vi "SingleGUI-Intravital.vi"() -> ()   [LabVIEW 2011]
uses:
  <vilib>/event_ctls.llb/lveventtype.ctl
  <vilib>/Utility/inputDevices.llb/mouseAcquire.vi
  <vilib>/Utility/inputDevices.llb/closeMouse.vi
panel:
  in  "Shutter":bool
  in  "LaserPower mW":dbl(slide) scale=1.0..500.0
  in  "Menu":string
  in  "Intensity":dbl(slide) scale=0.0..5.0
  in  "PMT2 ON":bool=TRUE caption="PMT2"
  in  "High Voltage PMT / V 2":u16(slide) caption="High Voltage PMT2 / V" max=1250 step=1 scale=0.0..1250.0
  in  "Pos [mm]":cluster{"x":dbl, "y":dbl}={"x"=56.550000000000004, "y"=34.7} {"x" min=-200.0 max=200.0 step=0.01 format="%.4f"; "y" min=-100.0 max=100.0 step=0.01 format="%.4f"}
  in  "Stage control":enum32{"xy", "Setup", "Status"}(tab)
  in  "Stepsize [mm]":dbl(slide)=0.4602583962404807 scale=0.01..5.0
  in  "Cluster":T1
  in  "clockwise":bool=TRUE
  in  "xy Angle":dbl
  in  "Objektiv Offsets":cluster{"x":dbl, "y":dbl, "z":dbl}[](array[cluster]) {"z" format="%#.3p"; "y" format="%#.3p"; "x" format="%#.3p"}
  out "scroll units^3":dbl
  out "Mouse inside?":T2
  out "scroll timed out":bool=TRUE
  out "endGUI":bool
  in  "z[mm]":dbl(slide) min=0.0 max=21.5 step=1e-05 scale format="%#.3f"
  in  "PMT Filter":sgl(ring) caption="filter.f1" items=["Split562", "Split495", "empty"]
  in  "Epi Filter":sgl(ring) caption="filter.f2" items=["emty"=0, "empty"=5]
  in  "PMT1 ON":bool=TRUE caption="PMT1"
  in  "High Voltage PMT / V":u16(slide) max=1250 step=1 scale=0.0..1250.0
  in  "stop 2":bool
  in  "continous":bool
  in  "LED":bool
  in  "single":bool
  in  "Camera Exposure (s)":dbl(slide)=0.08565902153685491 min=1e-06 step=0.001 scale=0.001..10.0 scale format="%#.3p"
  in  "Channel1=f":bool
  in  "End Program":bool
  out "Image":T3(plugin-control)
  in  "Detector":u16(ring)
  out "Image Nr":i32
  in  "Conversion Method":u32(ring)=2 items=["Full Dynamic"=0, "Given Range"=2, "90% Dynamic"=3, "Given Percent Range"=4]
  in  "Max. Value":i32=1000 min=1 max=64000 step=50
  in  "Min. Value":i32 min=0 max=32000 step=10
  # "Colibri Laser Scanning                                                                                                                                                 TILL Photonics GmbH"
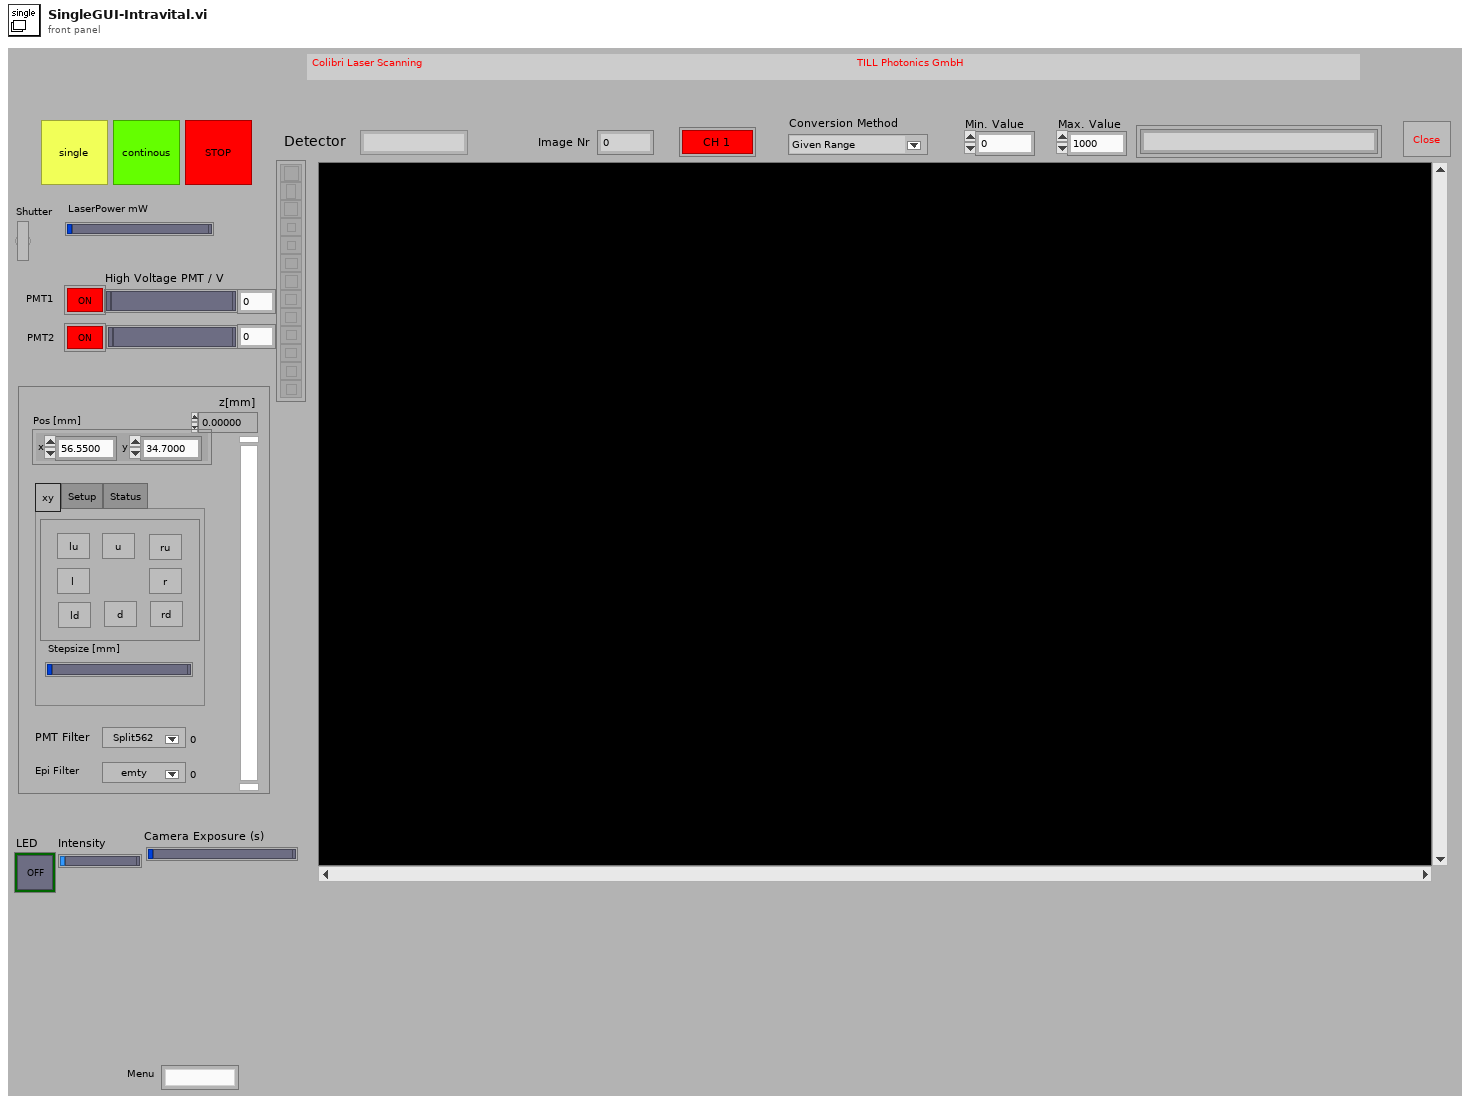
[diagram p1: front panel]
types:
  T1 = cluster{"r":bool, "ru":bool, "u":bool, "lu":bool, "l":bool, "ld":bool, "d":bool, "rd":bool}
  T2 = typedef "lveventtype.ctl" = enum32{"Null", "Timeout", "App Instance Close", "App Instance Close?", "Autoscale Range Change", "Cell Edit", "Cell Edit?", "Cursor Grab", "Cursor Grab?", "Cursor Move", "Cursor Release", "Data Change", "Direction Change", "Display State Change", "Drag Ended", "Drag Enter", "Drag Leave", "Drag Over", "Drag Source Update", "Drag Starting", "Drag Starting?", "Drop", "Exec State Change", "Key Down", "Key Down?", "Key Repeat", "Key Repeat?", "Key Up", "Listbox Double Click", "Menu Activation?", "Menu Selection (App)", "Menu Selection? (App)", "Menu Selection (User)", "Mouse Down", "Mouse Down?", "Mouse Enter", "Mouse Leave", "Mouse Move", "Mouse Up", "NI Security User Change (App)", "Pane Size", "Panel Close", "Panel Close?", "Panel Resize", "Plot Attribute Change", "Scale Range Change", "Shortcut Menu Activation?", "Shortcut Menu Selection (App)", "Shortcut Menu Selection? (App)", "Shortcut Menu Selection (User)", "Tree Double Click", "Tree Drag", "Tree Drag?", "Tree Drop", "Tree Drop?", "Tree Item Close", "Tree Item Close?", "Tree Item Open", "Tree Item Open?", "Value Change"}
  T3 = typedef "IMAQ Image.ctl" = refnum<image>
  T4 = enum16{"None/#Datasets", "Clear", "TagValueOf#", "AddValues", "ReadValue", "ChangeValue", "Get all"}
  T5 = enum16{"status", "createIMAQ", "getIMAQ", "getNumber", "deleteIMAQ", "deleteAll", "MemoryUsage", "GetAccess", "DecreaseAccess", "ActualIndex", "ElementToNumber"}
  T6 = cluster{"default value 1":dbl, "default value 1":dbl, "default value 1":dbl}
  T7 = cluster{"menu tag":string, "menu-vi":refnum<vi>}[]
  T8 = cluster{"Horizontal":i32, "Vertical":i32, "Scrolling":i32}
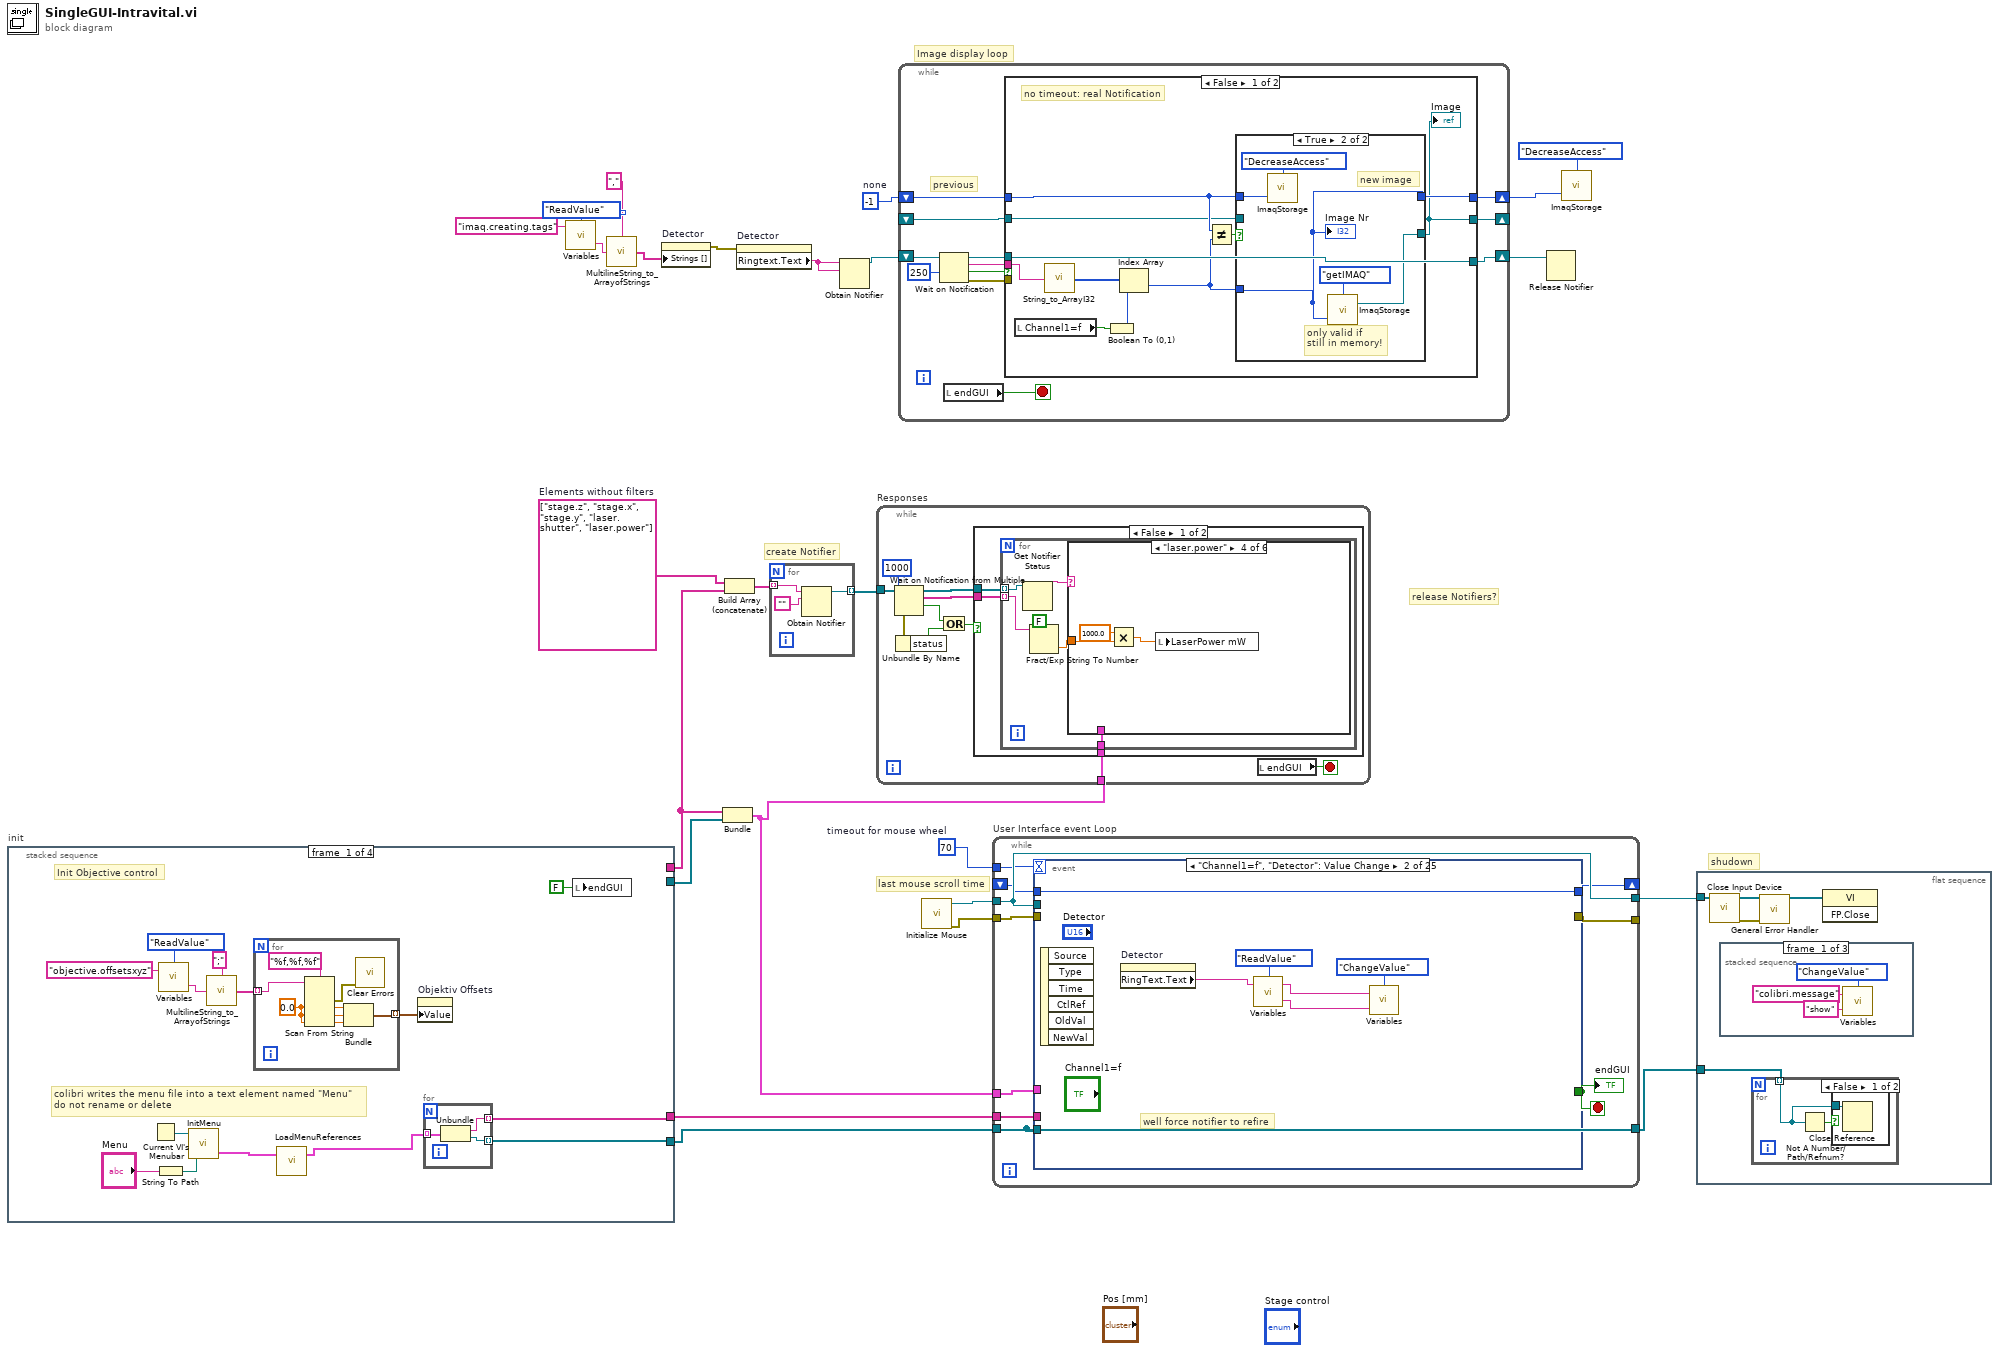
[diagram p0: block diagram]
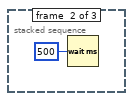
[diagram p2: hidden frame]
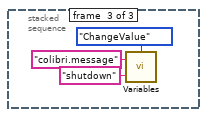
[diagram p3: hidden frame]
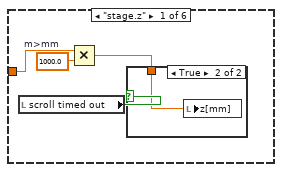
[diagram p5: hidden frame]
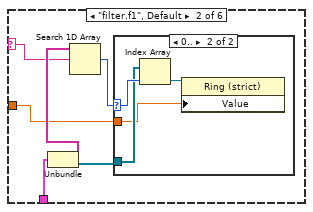
[diagram p7: hidden frame]
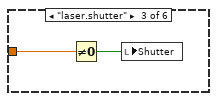
[diagram p9: hidden frame]
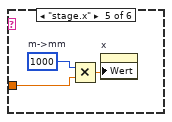
[diagram p10: hidden frame]
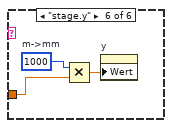
[diagram p11: hidden frame]
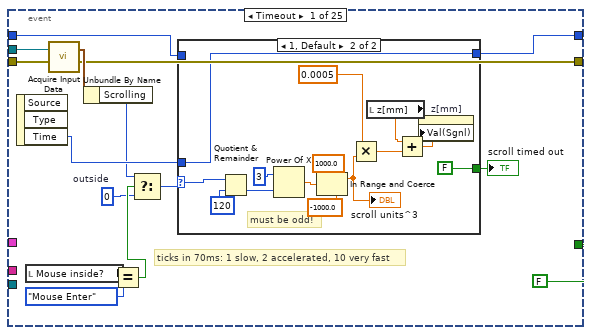
[diagram p13: hidden frame]
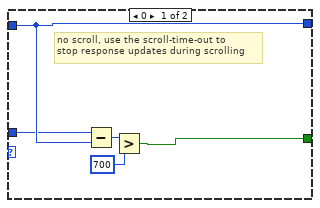
[diagram p14: hidden frame]
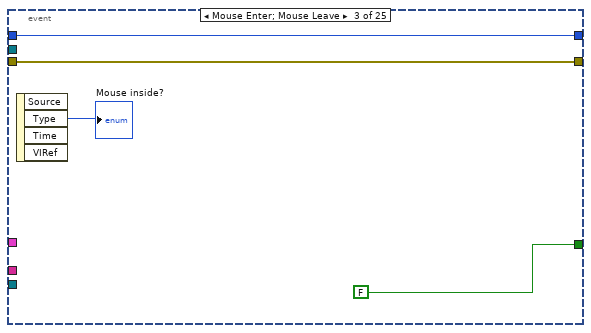
[diagram p15: hidden frame]
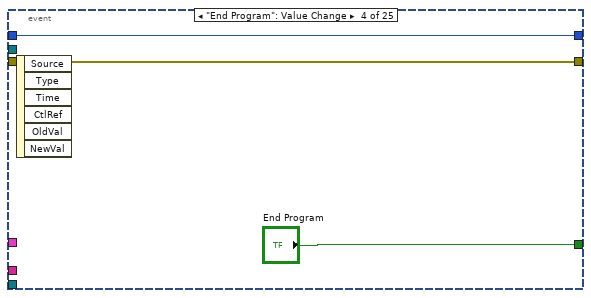
[diagram p16: hidden frame]
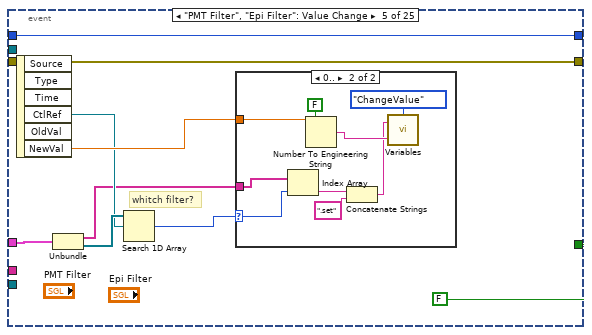
[diagram p17: hidden frame]
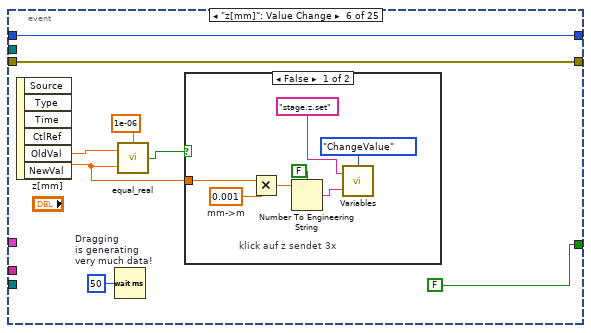
[diagram p19: hidden frame]
diagram:
  w5 = u32 70  # timeout for mouse wheel
  w13 = string[] ["stage.z", "stage.x", "stage.y", "laser.shutter", "laser.power"]  # Elements without filters
  w22 = -1  # none
  # "Image display loop"
  # "shudown"
  # "last mouse scroll time"
  # "release Notifiers?"
  # "create Notifier"
  n1 = stacked-sequence "init" {
    tunnel: [_ w55 _ _] -> w11
    tunnel: [_ w54 _ _] -> w9
    tunnel: [w27 _ _ _] -> w4
    tunnel: [w26 _ _ _] -> w3
    frame #0 {
      # "colibri writes the menu file into a text element named \"Menu\"\ndo not rename or delete"
      # "Init Objective control"
      n2 = Current VI's Menubar() -> (w32:refnum<k9>)
      n3 = String To Path(string="Menu") -> (path=w30:path)
      n4 = call "Variables.vi"("Tag in"="objective.offsetsxyz", "Command"=T4."ReadValue") -> ("value out"=w36:string)  [unwired: 1 in, 2 out]
      n5 = call "InitMenu.vi"("menu-ini"=w30, "menubar"=w32) -> ("Menu-VI"=w31:cluster{"item tag":string, "vi-Path":path}[])  [unwired: 1 out]
      n6 = call "MultilineString_to_ArrayofStrings.vi"("String 1"=w36, "NewLineString"=";") -> ("String Array"=w35:string[])
      n7 = for {
        tunnel: w35 -> [w44] mode=indexing
        tunnel: [w43] -> w34 mode=indexing
        w46 = 0.0 ("default value 1")
        n8 = Scan From String(format string="%f,%f,%f" ("Format-String"), input string=w44, default 1=w46, default 2=w46, default 3=w46) -> (error out=w45:errorcluster, output 1=w49:dbl, output 2=w48:dbl, output 3=w47:dbl)  [unwired: 2 in, 2 out]
        n9 = Bundle("default value 1"=w49, "default value 1"=w48, "default value 1"=w47) -> (w43:T6)  [unwired: 1 out]
        n10 = call <vilib>:"Clear Errors.vi"("error in (no error)"=w45) -> ()  [unwired: 7 out]
      }
      n11 = call "LoadMenuReferences.vi"("Menu-VI"=w31) -> ("Menu"=w28:T7)  [unwired: 1 in, 1 out]
      n12 = property on="Objektiv Offsets" class="Arr (strict)"("Value"=w34) -> ()  [unwired: 2 in, 2 out]
      n13 = for {
        tunnel: w28 -> [w42] mode=indexing
        tunnel: [w41] -> w27 mode=indexing
        tunnel: [w40] -> w26 mode=indexing
        n14 = Unbundle(w42) -> ("menu tag"=w41:string, "menu-vi"=w40:refnum<vi>)
      }
      n15 = local write "endGUI"(FALSE ("stop 2")) -> ()
    }
    frame #1 {
      # "Init filter slider control"
      n16 = call "Variables.vi"("Tag in"="filter.tags", "Command"=T4."ReadValue") -> ("value out"=w57:string)  [unwired: 1 in, 2 out]
      n17 = call "MultilineString_to_ArrayofStrings.vi"("String 1"=w57, "NewLineString"=",") -> ("String Array"=w55:string[])
      n18 = control-ref of="Epi Filter"() -> (w53:refnum<vi>)
      n19 = control-ref of="PMT Filter"() -> (w52:refnum<vi>)
      n20 = Build Array(w52, w53) -> (w51:refnum<vi>[])
      n21 = for {
        tunnel: w55 -> [w63] mode=indexing
        tunnel: w51 -> [w61] mode=indexing
        tunnel: [w60] -> w54 mode=indexing
        n22 = Concatenate Strings(w63, ".label" ("string")) -> (w64:string)
        n23 = call "Variables.vi"("Tag in"=w64, "Command"=T4."ReadValue") -> ("value out"=w68:string)  [unwired: 1 in, 2 out]
        n24 = call "MultilineString_to_ArrayofStrings.vi"("String 1"=w68, "NewLineString"=";") -> ("String Array"=w67:string[])
        n25 = for {
          tunnel: w67 -> [w77] mode=indexing
          tunnel: [w72] -> w66 mode=indexing
          n26 = call "SplitAtLast.vi"("search char"=",", "In-String"=w77) -> ("end"=w75:string, "Front (default)"=w74:string)
          n27 = Fract/Exp String To Number(use system decimal point (T)=FALSE, string=w75) -> (number=w73:dbl)  [unwired: 3 out]
          n28 = Bundle("Front (default)"=w74, w73) -> (w72:cluster{"Front (default)":string, dbl})  [unwired: 1 out]
        }
        n29 = property on="Property Node" class="Ring (strict)"(reference=w61, "StringsAndValues[]"=w66, "Visible"=TRUE, "Caption.Text"=w63) -> (reference out=w60:refnum<vi>)  [unwired: 1 in, 1 out]
      }
    }
    frame #2 {
      # "it would be good to Read/update all elements"
      # "update obj.mag\nan external change in Objective.set will probably forget to set obj.mag?"
      n30 = call "Variables.vi"("Tag in"="stage.z", "Command"=T4."ReadValue") -> ("value out"=w82:string)  [unwired: 1 in, 2 out]
      n31 = call "Variables.vi"("Tag in"="obj.mag", "Command"=T4."ReadValue") -> ("value out"=w86:string)  [unwired: 1 in, 2 out]
      n32 = Fract/Exp String To Number(use system decimal point (T)=TRUE, string=w82) -> (number=w81:dbl)  [unwired: 3 out]
      n33 = Decimal String To Number(string=w86, default (0L)=60 ("default (0 I32)")) -> ()  [unwired: 3 out]
      n34 = Multiply(x=1000.0, y=w81) -> (x*y=w79:dbl)
      n35 = local write "z[mm]"(w79) -> ()
    }
    frame #3 {
      n36 = property on="Image" class="ImageControl"() -> ("16-bit Display Conversion Method"=w92:u32)  [unwired: 2 in, 2 out]
      n37 = local write "Conversion Method"(w92) -> ()
      n38 = call "Variables.vi"("value"="hide", "Tag in"="colibri.message", "Command"=T4."ChangeValue") -> ()  [unwired: 3 out]
    }
  }
  n39 = call "Variables.vi"("Tag in"="imaq.creating.tags", "Command"=T4."ReadValue") -> ("value out"=w17:string)  [unwired: 1 in, 2 out]
  n40 = call "MultilineString_to_ArrayofStrings.vi"("String 1"=w17, "NewLineString"=",") -> ("String Array"=w15:string[])
  n41 = property on="Detector" class="Ring (strict)"("Strings []"=w15) -> (error out=w14:errorcluster)  [unwired: 2 in, 1 out]
  n42 = Bundle("String Array"=w11, w9) -> (w10:cluster{"String Array":string[], refnum<vi>[]})  [unwired: 1 out]
  n43 = Build Array (concatenate)(w13, w11) -> (w12:string[])
  n44 = property on="Detector" class="Ring (strict)"(error in=w14) -> ("Ringtext.Text"=w23:string)  [unwired: 1 in, 2 out]
  n45 = for {
    tunnel: w12 -> [w94] mode=indexing
    tunnel: [w95] -> w8 mode=indexing
    n46 = Obtain Notifier(name (unnamed)=w94, notification data type="") -> (notifier out=w95:refnum<notifier>)  [unwired: 2 in, 2 out]
  }
  n47 = Obtain Notifier(name (unnamed)=w23, notification data type=w23) -> (notifier out=w25:refnum<notifier>)  [unwired: 2 in, 2 out]
  n48 = while "Responses" {
    tunnel: w8 -> [w105]
    tunnel: w10 -> [w97]
    stop <- w96 stop-if-true
    n49 = Wait on Notification from Multiple(0:w105, 2:1000 ("timeout in ms (-1)")) -> (8:w100:refnum<notifier>[], 9:w99:string[], 10:w101:bool, 11:w103:errorcluster)  [unwired: 1 in, 1 out]
    n50 = Unbundle By Name(w103) -> ("status"=w102:bool)
    n51 = Or(x=w101, y=w102) -> (x .or. y?=w98:bool)
    n52 = case shown="False" w98 {
      tunnel: w100 -> [w108 _]
      tunnel: w99 -> [w107 _]
      tunnel: w97 -> [w106 _]
      frame False {
        n53 = for {
          tunnel: w108 -> [w114] mode=indexing
          tunnel: w107 -> [w112] mode=indexing
          tunnel: w106 -> [w109]
          n54 = Get Notifier Status(notifier=w114) -> (notifier name=w113:string)  [unwired: 1 in, 4 out]
          n55 = Fract/Exp String To Number(use system decimal point (T)=FALSE, string=w112) -> (number=w110:dbl)  [unwired: 3 out]
          n56 = case shown="\"laser.power\"" w113 {
            selector: w113 -> [_ w122 _ _ _ _]
            tunnel: w110 -> [w118 w120 w130 w134 w136 w140]
            tunnel: w109 -> [_ w125 _ _ _ _]
            frame "stage.z" {
              w116 = 1000.0  # m>mm
              n57 = local read "scroll timed out"() -> (w115:bool)
              n58 = Multiply(x=w118, y=w116) -> (x*y=w117:dbl)
              n59 = case shown="True" w115 {
                tunnel: w117 -> [_ w119]
                frame False {
                }
                frame True {
                  n60 = local write "z[mm]"(w119) -> ()
                }
              }
            }
            frame "filter.f1", Default {
              n61 = Unbundle(w125) -> ("String Array"=w123:string[], w124:refnum<vi>[])
              n62 = Search 1D Array(1D array=w123, element=w122) -> (index of element=w121:i32)  [unwired: 1 out]
              n63 = case shown="0.." w121 {
                selector: w121 -> [_ w129]
                tunnel: w124 -> [_ w128]
                tunnel: w120 -> [_ w126]
                frame -1, Default {
                }
                frame 0.. {
                  n64 = Index Array(array=w128, index=w129) -> (element=w127:refnum<vi>)
                  n65 = property on="Property Node" class="Ring (strict)"(reference=w127, "Value"=w126) -> ()  [unwired: 1 in, 2 out]
                }
              }
            }
            frame "laser.shutter" {
              n66 = Not Equal To 0?(x=w130) -> (x != 0?=w131:bool)
              n67 = local write "Shutter"(w131) -> ()
            }
            frame "laser.power" {
              n68 = Multiply(x=1000.0, y=w134) -> (x*y=w132:dbl)
              n69 = local write "LaserPower mW"(w132) -> ()
            }
            frame "stage.x" {
              w137 = 1000  # m->mm
              n70 = Multiply(x=w137, y=w136) -> (x*y=w135:dbl)
              n71 = property on="x" class="DigNum (strict)"("Wert"=w135) -> ()  [unwired: 2 in, 2 out]
            }
            frame "stage.y" {
              w139 = 1000  # m->mm
              n72 = Multiply(x=w139, y=w140) -> (x*y=w138:dbl)
              n73 = property on="y" class="DigNum (strict)"("Wert"=w138) -> ()  [unwired: 2 in, 2 out]
            }
          }
        }
      }
      frame True {
        # "err or timeout"
      }
    }
    n74 = local read "endGUI"() -> (w96:bool)
  }
  n75 = while {
    shift-right: [w149] -> w21
    shift-left: w22 -> [w150]
    shift-right: [w144] -> w24
    shift-left: w25 -> [w152]
    shift-right: [w143] -> _
    shift-left: _ -> [w142]
    stop <- w141 stop-if-true
    # "previous"
    n76 = Wait on Notification(notifier=w152, timeout in ms (-1)=250) -> (notifier out=w145:refnum<notifier>, notification=w151:string, timed out?=w147:bool, error out=w148:errorcluster)  [unwired: 1 in, 1 out]
    n77 = local read "endGUI"() -> (w141:bool)
    n78 = case shown="False" w147 {
      tunnel: w151 -> [w157 _]
      tunnel: w150 -> [w162 w178]
      tunnel: [w159 w178] -> w149
      tunnel: w148 -> [_ _]
      tunnel: w145 -> [w163 w177]
      tunnel: [w163 w173] -> w144
      tunnel: [w158 w171] -> w143
      tunnel: w142 -> [w160 w171]
      frame False {
        # "no timeout: real Notification"
        n79 = local read "Channel1=f"() -> (w153:bool)
        n80 = call "String_to_ArrayI32.vi"("String"=w157) -> ("ArrayI32"=w154:i32[])  [unwired: 1 in]
        n81 = Boolean To (0,1)(Boolean=w153) -> (0, 1=w156:i16)
        n82 = Index Array(array=w154, index=w156) -> (element=w155:i32)
        n83 = Not Equal?(x=w162, y=w155) -> (x != y?=w161:bool)
        n84 = case shown="True" w161 {
          tunnel: [w165 w170] -> w158
          tunnel: w155 -> [_ w166]
          tunnel: w162 -> [w164 w169]
          tunnel: w160 -> [w165 _]
          tunnel: [w164 w166] -> w159
          frame False {
            # "new data, same image"
          }
          frame True {
            # "only valid if\nstill in memory!"
            # "new image"
            n85 = call "ImaqStorage.vi"("Number"=w169, "Command"=T5."DecreaseAccess") -> ()  [unwired: 1 in, 2 out]
            n86 = call "ImaqStorage.vi"("Number"=w166, "Command"=T5."getIMAQ") -> ("IMAQ out"=w170:T3)  [unwired: 1 in, 1 out]
            "Image Nr" <- w166
          }
        }
        "Image" <- w158
      }
      frame True {
        # "time out\ngood for checking the stop button\nis there a new \"link to\"?"
        n87 = property on="Detector" class="Ring (strict)"() -> ("Ringtext.Text"=w172:string)  [unwired: 2 in, 2 out]
        n88 = Get Notifier Status(notifier=w177) -> (notifier out=w174:refnum<notifier>, notifier name=w176:string)  [unwired: 1 in, 3 out]
        n89 = Not Equal?(x=w172, y=w176) -> (x != y?=w175:bool)
        n90 = case shown="True" w175 {
          tunnel: w174 -> [w179 w182]
          tunnel: [w179 w181] -> w173
          tunnel: w172 -> [_ w180]
          frame False {
            # "same as before"
          }
          frame True {
            n91 = Release Notifier(notifier=w182) -> ()  [unwired: 1 in, 4 out]
            n92 = Obtain Notifier(name (unnamed)=w180, notification data type=w180) -> (notifier out=w181:refnum<notifier>)  [unwired: 2 in, 2 out]
          }
        }
      }
    }
  }
  n93 = call <vilib>:"Initialize Mouse.vi"() -> ("error out"=w6:errorcluster, "device ID"=w7:refnum<k1>)  [unwired: 1 in, 9 out]
  n94 = while "User Interface event Loop" {
    tunnel: w10 -> [w192]
    tunnel: w7 -> [w191]
    tunnel: [w191] -> w2
    tunnel: w6 -> [w190]
    tunnel: [w189] -> _
    shift-right: [w187] -> _
    shift-left: _ -> [w188]
    tunnel: w5 -> [w185]
    tunnel: w4 -> [w184]
    tunnel: w3 -> [w183]
    tunnel: [w183] -> w1
    stop <- w186 stop-if-true
    n95 = event shown="[1] \"Channel1=f\", \"Detector\": Value Change" {
      selector: _ -> [_ _ _ _ _ _ _ _ _ _ _ _ _ _ _ _ _ _ _ _ _ _ _ _ _]
      dyn-events: _ -> [_ _ _ _ _ _ _ _ _ _ _ _ _ _ _ _ _ _ _ _ _ _ _ _ _]
      timeout: w185 -> [_ _ _ _ _ _ _ _ _ _ _ _ _ _ _ _ _ _ _ _ _ _ _ _ _]
      tunnel: [FALSE ("stop") _ FALSE ("stop") "End Program" FALSE FALSE FALSE FALSE ("stop") FALSE ("stop") FALSE ("stop") _ _ _ _ _ _ _ _ FALSE ("stop") FALSE ("stop") _ _ _ w467 w480] -> w186
      tunnel: w192 -> [_ _ _ _ w246 _ _ _ _ _ _ _ _ _ _ _ _ _ _ _ _ _ _ _ _]
      tunnel: w191 -> [w207 _ _ _ _ _ _ _ _ _ _ _ _ _ _ _ _ _ _ _ _ _ _ _ _]
      tunnel: w190 -> [w206 _ w233 w237 w240 w258 w274 w283 w293 w332 w354 w365 w371 w382 w391 w397 w402 w410 w419 w431 w444 _ _ _ _]
      tunnel: [w199 _ w233 w237 w240 w258 w274 w283 w293 w332 w354 w365 w371 w382 w391 w397 w402 w410 w419 w431 w444 _ _ _ _] -> w189
      tunnel: w188 -> [w203 w232 w234 w238 w241 w259 w273 w284 w294 w331 w355 w366 w372 w383 w392 w398 w403 w411 w420 w432 w450 w451 w459 w466 w479]
      tunnel: [w204 w232 w234 w238 w241 w259 w273 w284 w294 w331 w355 w366 w372 w383 w392 w398 w403 w411 w420 w432 w450 w451 w459 w466 w479] -> w187
      tunnel: w184 -> [_ _ _ _ _ _ _ _ _ _ _ _ _ _ _ _ _ _ _ _ _ _ _ w469 _]
      tunnel: w183 -> [_ _ _ _ _ _ _ _ _ _ _ _ _ _ _ _ _ _ _ _ _ _ _ w468 _]
      event Timeout {
        w193 = 0  # outside
        # "ticks in 70ms: 1 slow, 2 accelerated, 10 very fast"
        n96 = event-data() -> ("Time"=w202:u32)  [unwired: 3 out]
        n97 = local read "Mouse inside?"() -> (w198:T2)
        n98 = call-poly <vilib>:"Acquire Input Data.vi"("device ID"=w207, "error in (no error)"=w206) -> ("axis info"=w205:T8, "error out"=w199:errorcluster)  [unwired: 1 in, 15 out]
        n99 = Unbundle By Name(w205) -> ("Scrolling"=w195:i32)
        n100 = Equal?(x=w198, y=lveventtype."Mouse Enter" ("Type")) -> (x = y?=w196:bool)
        n101 = Select(t=w195, s=w196, f=w193) -> (s? t:f=w194:i32)
        n102 = case shown="1, Default" w194 {
          selector: w194 -> [_ w222]
          tunnel: w203 -> [w212 _]
          tunnel: [w212 w223] -> w204
          tunnel: w202 -> [w209 w223]
          tunnel: [w208 FALSE] -> w200
          frame 0 {
            # "no scroll, use the scroll-time-out to\nstop response updates during scrolling"
            n103 = Subtract(x=w209, y=w212) -> (x-y=w211:u32)
            n104 = Greater?(x=w211, y=u32 700) -> (0:w208:bool)
          }
          frame 1, Default {
            # "must be odd!"
            n105 = Quotient & Remainder(x=w222, y=120) -> (floor(x/y)=w220:i32)  [unwired: 1 out]
            n106 = Power Of X(1:w220, 2:3 ("y")) -> (0:w218:dbl)
            n107 = In Range and Coerce(upper limit=1000.0, x=w218, lower limit=-1000.0) -> (coerced(x)=w217:dbl)  [unwired: 1 out]
            "scroll units^3" <- w217
            n108 = Multiply(x=0.0005 ("min.step"), y=w217) -> (x*y=w226:dbl)
            n109 = local read "z[mm]"() -> (w225:dbl)
            n110 = Add(x=w225, y=w226) -> (x+y=w224:dbl)
            n111 = property on="z[mm]" class="Slide (strict)"("Val(Sgnl)"=w224) -> ()  [unwired: 2 in, 2 out]
          }
        }
        "scroll timed out" <- w200
      }
      event "Channel1=f", "Detector": Value Change {
        # "well force notifier to refire"
        n112 = event-data() -> ()  [unwired: 7 out]
        n113 = property on="Detector" class="Ring (strict)"() -> ("RingText.Text"=w229:string)  [unwired: 2 in, 2 out]
        n114 = call "Variables.vi"("Tag in"=w229, "Command"=T4."ReadValue") -> ("value out"=w227:string, "Tag out"=w228:string)  [unwired: 1 in, 1 out]
        n115 = call "Variables.vi"("value"=w227, "Tag in"=w228, "Command"=T4."ChangeValue") -> ()  [unwired: 3 out]
      }
      event Mouse Enter; Mouse Leave {
        n116 = event-data() -> ("Type"=→"Mouse inside?":T2)  [unwired: 4 out]
      }
      event "End Program": Value Change {
        n117 = event-data() -> ()  [unwired: 7 out]
      }
      event "PMT Filter", "Epi Filter": Value Change {
        # "whitch filter?"
        n118 = event-data() -> ("CtlRef"=w244:refnum<vi>, "NewVal"=w248:sgl)  [unwired: 5 out]
        n119 = Unbundle(w246) -> ("String Array"=w242:string[], w245:refnum<vi>[])
        n120 = Search 1D Array(1D array=w245, element=w244) -> (index of element=w243:i32)  [unwired: 1 out]
        n121 = case shown="0.." w243 {
          selector: w243 -> [_ w252]
          tunnel: w248 -> [_ w257]
          tunnel: w242 -> [_ w253]
          frame -1, Default {
          }
          frame 0.. {
            n122 = Index Array(array=w253, index=w252) -> (element=w251:string)
            n123 = Number To Engineering String(1:FALSE ("use system decimal point (T)"), 4:w257) -> (0:w256:string)  [unwired: 2 out]
            n124 = Concatenate Strings(w251, ".set" ("string")) -> (w250:string)
            n125 = call "Variables.vi"("value"=w256, "Tag in"=w250, "Command"=T4."ChangeValue") -> ()  [unwired: 3 out]
          }
        }
      }
      event "z[mm]": Value Change {
        w264 = u32 50  # Dragging is generating very much data!
        n126 = event-data() -> ("OldVal"=w263:dbl, "NewVal"=w262:dbl)  [unwired: 5 out]
        n127 = Wait (ms)(milliseconds to wait=w264) -> ()  [unwired: 1 out]
        n128 = call "equal_real.vi"("max rel deviation"=1e-06, "b"=w262, "a"=w263) -> ("Equal"=w261:bool)
        n129 = case shown="False" w261 {
          tunnel: w262 -> [w267 _]
          frame False {
            w272 = 0.001  # mm->m
            # "klick auf z sendet 3x"
            n130 = Multiply(x=w267, y=w272) -> (x*y=w271:dbl)
            n131 = Number To Engineering String(1:FALSE ("use system decimal point (T)"), 4:w271) -> (0:w269:string)  [unwired: 2 out]
            n132 = call "Variables.vi"("value"=w269, "Tag in"="stage.z.set", "Command"=T4."ChangeValue") -> ()  [unwired: 3 out]
          }
          frame True {
          }
        }
      }
      event "Pos [mm].x": Value Change {
        w281 = 0.001  # mm->m
        n133 = event-data() -> ("NewVal"=w279:dbl)  [unwired: 6 out]
        n134 = Multiply(x=w279, y=w281) -> (x*y=w282:dbl)
        n135 = Number To Fractional String(use system decimal point (T)=FALSE, number=w282) -> (F-format string=w277:string)  [unwired: 2 out]
        n136 = call "Variables.vi"("value"=w277, "Tag in"="stage.x.set" ("Tag"), "Command"=T4."ChangeValue") -> ()  [unwired: 3 out]
      }
      event "Pos [mm].y": Value Change {
        w291 = 0.001  # mm->m
        n137 = event-data() -> ("NewVal"=w286:dbl)  [unwired: 6 out]
        n138 = Multiply(x=w286, y=w291) -> (x*y=w292:dbl)
        n139 = Number To Fractional String(use system decimal point (T)=FALSE, number=w292) -> (F-format string=w289:string)  [unwired: 2 out]
        n140 = call "Variables.vi"("value"=w289, "Tag in"="stage.y.set" ("Tag"), "Command"=T4."ChangeValue") -> ()  [unwired: 3 out]
      }
      event "Cluster": Value Change {
        w309 = 0.001  # mm->m
        # "anordung: index*45=winkel!"
        n141 = event-data() -> ("OldVal"=w325:T1)  [unwired: 6 out]
        n142 = Not Equal?(x=w325, y="Cluster") -> (x != y?=w324:T1)
        n143 = Cluster To Array(cluster=w324) -> (array=w323:bool[])
        n144 = Select(t=-1.0, s="clockwise", f=1.0) -> (s? t:f=w298:dbl)
        n145 = Search 1D Array(1D array=w323, element=TRUE ("Element")) -> (index of element=w321:i32)  [unwired: 1 out]
        n146 = Multiply(x=45, y=w321) -> (x*y=w320:i32)
        n147 = Multiply(x=w320, y=w298) -> (x*y=w299:dbl)
        n148 = Divide(x=3.141592653589793, y=180.0) -> (x/y=w300:dbl)
        n149 = Add(x=w299, y="xy Angle") -> (x+y=w297:dbl)
        n150 = Multiply(x=w297, y=w300) -> (x*y=w307:dbl)
        n151 = local read "Pos [mm]"() -> (w314:cluster{"x":dbl, "y":dbl})
        n152 = Cosine(x=w307) -> (cos(x)=w317:dbl)
        n153 = Sine(x=w307) -> (sin(x)=w316:dbl)
        n154 = Build Array(w317, w316) -> (w315:dbl[])
        n155 = Cluster To Array(cluster=w314) -> (array=w313:dbl[])
        n156 = Multiply(x=w315, y="Stepsize [mm]") -> (x*y=w318:dbl[])
        n157 = Add(x=w318, y=w313) -> (x+y=w311:dbl[])
        n158 = Multiply(x=w309, y=w311) -> (x*y=w310:dbl[])
        n159 = for {
          tunnel: w310 -> [w326] mode=indexing
          tunnel: string[] ["stage.x.set", "stage.y.set"] -> [w327] mode=indexing
          n160 = Number To Fractional String(use system decimal point (T)=FALSE, number=w326) -> (F-format string=w330:string)  [unwired: 2 out]
          n161 = call "Variables.vi"("value"=w330, "Tag in"=w327, "Command"=T4."ChangeValue") -> ()  [unwired: 3 out]
        }
      }
      event "Objektiv Offsets": Value Change {
        # "Obsolete??"
        n162 = event-data() -> ("OldVal"=w334:cluster{"x":dbl, "y":dbl, "z":dbl}[], "NewVal"=w333:cluster{"x":dbl, "y":dbl, "z":dbl}[])  [unwired: 5 out]
        n163 = for {
          tunnel: w334 -> [w339] mode=indexing
          tunnel: w333 -> [w337] mode=indexing
          i -> [w336]
          n164 = Not Equal?(x=w339, y=w337) -> (x != y?=w338:bool)
          n165 = case shown="True" w338 {
            tunnel: w337 -> [_ w350]
            tunnel: w336 -> [_ w345]
            frame False {
            }
            frame True {
              n166 = Unbundle(w350) -> ("x"=w349:dbl, "y"=w348:dbl, "z"=w347:dbl)
              n167 = Number To Decimal String(number=w345) -> (decimal integer string=w344:string)  [unwired: 1 out]
              n168 = Format Into String(format string="%f,%f,%f" ("Format-String"), w349, w348, w347) -> (resulting string=w341:string)  [unwired: 2 in, 1 out]
              n169 = Concatenate Strings("obj.offsetxyz." ("Tag in"), w344) -> (w342:string)
              n170 = call "Variables.vi"("value"=w341, "Tag in"=w342, "Command"=T4."ChangeValue") -> ()  [unwired: 3 out]
            }
          }
        }
      }
      event "Camera Exposure (s)": Value Change {
        n171 = event-data() -> ()  [unwired: 7 out]
        n172 = property on="Detector" class="Ring (strict)"() -> ("RingText.Text"=w352:string)  [unwired: 2 in, 2 out]
        n173 = Search/Split String(string=w352, search string/char (-)="." ("Nach String/Zeichen suchen (-)")) -> (substring before match=w351:string)  [unwired: 3 out]
        n174 = Number To Fractional String(use system decimal point (T)=FALSE, number="Camera Exposure (s)") -> (F-format string=w358:string)  [unwired: 2 out]
        n175 = Concatenate Strings(w351, ".exposure" ("Tag in")) -> (w361:string)
        n176 = call "Variables.vi"("value"=w358, "Tag in"=w361, "Command"=T4."ChangeValue") -> ()  [unwired: 3 out]
      }
      event "single": Value Change {
        n177 = event-data() -> ()  [unwired: 7 out]
        n178 = property on="Detector" class="Ring (strict)"() -> ("RingText.Text"=w363:string)  [unwired: 2 in, 2 out]
        n179 = Search/Split String(string=w363, search string/char (-)="." ("Nach String/Zeichen suchen (-)")) -> (substring before match=w362:string)  [unwired: 3 out]
        n180 = Concatenate Strings(w362, ".number.set" ("notification")) -> (w369:string)
        n181 = call "Variables.vi"("value"="1" ("notification"), "Tag in"=w369, "Command"=T4."ChangeValue") -> ()  [unwired: 3 out]
      }
      event "LED": Value Change {
        n182 = event-data() -> ()  [unwired: 7 out]
        n183 = Select(t="1" ("value"), s="LED", f="0") -> (s? t:f=w377:string)
        n184 = call "Variables.vi"("value"=w377, "Tag in"="led.set", "Command"=T4."ChangeValue") -> ()  [unwired: 3 out]
      }
      event "continous": Value Change {
        n185 = event-data() -> ()  [unwired: 7 out]
        n186 = property on="Detector" class="Ring (strict)"() -> ("RingText.Text"=w380:string)  [unwired: 2 in, 2 out]
        n187 = Search/Split String(string=w380, search string/char (-)="." ("Nach String/Zeichen suchen (-)")) -> (substring before match=w379:string)  [unwired: 3 out]
        n188 = Concatenate Strings(w379, ".number.set" ("notification")) -> (w387:string)
        n189 = call "Variables.vi"("value"="100000" ("notification"), "Tag in"=w387, "Command"=T4."ChangeValue") -> ()  [unwired: 3 out]
      }
      event "stop 2": Value Change {
        n190 = event-data() -> ()  [unwired: 7 out]
        n191 = property on="Detector" class="Ring (strict)"() -> ("RingText.Text"=w389:string)  [unwired: 2 in, 2 out]
        n192 = Search/Split String(string=w389, search string/char (-)="." ("Nach String/Zeichen suchen (-)")) -> (substring before match=w388:string)  [unwired: 3 out]
        n193 = Concatenate Strings(w388, ".number.set" ("notification")) -> (w395:string)
        n194 = call "Variables.vi"("value"="0" ("notification"), "Tag in"=w395, "Command"=T4."ChangeValue") -> ()  [unwired: 3 out]
      }
      event "Min. Value", "Max. Value", "Conversion Method": Value Change {
        n195 = event-data() -> ()  [unwired: 7 out]
        n196 = property on="Image" class="ImageControl"("16-bit Display Conversion Method"="Conversion Method", "16-bit Display Maximum Value"="Max. Value", "16-bit Display Minimum Value"="Min. Value") -> ()  [unwired: 2 in, 2 out]
      }
      event "High Voltage PMT / V": Value Change {
        n197 = event-data() -> ("NewVal"=w404:u16)  [unwired: 6 out]
        n198 = local read "PMT1 ON"() -> (w405:bool)
        n199 = case shown="True" w405 {
          tunnel: w404 -> [_ w409]
          frame False {
          }
          frame True {
            n200 = Number To Decimal String(number=w409) -> (decimal integer string=w406:string)  [unwired: 1 out]
            n201 = call "Variables.vi"("value"=w406, "Tag in"="pmt.1.hv.set", "Command"=T4."ChangeValue") -> ()  [unwired: 3 out]
          }
        }
      }
      event "High Voltage PMT / V 2": Value Change {
        n202 = event-data() -> ("NewVal"=w412:u16)  [unwired: 6 out]
        n203 = local read "PMT2 ON"() -> (w413:bool)
        n204 = case shown="True" w413 {
          tunnel: w412 -> [_ w417]
          frame False {
          }
          frame True {
            n205 = Number To Decimal String(number=w417) -> (decimal integer string=w414:string)  [unwired: 1 out]
            n206 = call "Variables.vi"("value"=w414, "Tag in"="pmt.2.hv.set", "Command"=T4."ChangeValue") -> ()  [unwired: 3 out]
          }
        }
      }
      event "PMT1 ON": Value Change {
        n207 = event-data() -> ()  [unwired: 7 out]
        n208 = case shown="True" "PMT1 ON" {
          tunnel: ["0" w429] -> w424
          tunnel: [u8 0 ("Disabled") u8 1 ("Disabled")] -> w425
          frame False {
            # "send 0"
          }
          frame True {
            # "send"
            n209 = Number To Decimal String(number="High Voltage PMT / V") -> (decimal integer string=w429:string)  [unwired: 1 out]
          }
        }
        n210 = property on="High Voltage PMT / V" class="Slide (strict)"("Fill Style"=w425) -> ()  [unwired: 2 in, 2 out]
        n211 = call "Variables.vi"("value"=w424, "Tag in"="pmt.1.hv.set", "Command"=T4."ChangeValue") -> ()  [unwired: 3 out]
      }
      event "PMT2 ON": Value Change {
        n212 = event-data() -> ()  [unwired: 7 out]
        n213 = case shown="True" "PMT2 ON" {
          tunnel: ["0" w442] -> w437
          tunnel: [u8 0 ("Disabled") u8 1 ("Disabled")] -> w438
          frame False {
            # "send 0"
          }
          frame True {
            # "send"
            n214 = Number To Decimal String(number="High Voltage PMT / V 2") -> (decimal integer string=w442:string)  [unwired: 1 out]
          }
        }
        n215 = property on="High Voltage PMT / V 2" class="Slide (strict)"("Fill Style"=w438) -> ()  [unwired: 2 in, 2 out]
        n216 = call "Variables.vi"("value"=w437, "Tag in"="pmt.2.hv.set", "Command"=T4."ChangeValue") -> ()  [unwired: 3 out]
      }
      event "Intensity": Value Change {
        n217 = event-data() -> ()  [unwired: 7 out]
        n218 = Number To Fractional String(use system decimal point (T)=FALSE ("Systemdezimalzeichen verwenden (T)"), number="Intensity") -> (F-format string=w446:string)  [unwired: 2 out]
        n219 = call "Variables.vi"("value"=w446, "Tag in"="led.intensity.set", "Command"=T4."ChangeValue") -> ()  [unwired: 3 out]
      }
      event "LaserPower mW": Value Change {
        n220 = event-data() -> ()  [unwired: 7 out]
        n221 = Divide "in W"(x="LaserPower mW", y=1000.0) -> (x/y=w454:dbl)
        n222 = Number To Fractional String(use system decimal point (T)=FALSE ("Systemdezimalzeichen verwenden (T)"), number=w454) -> (F-format string=w456:string)  [unwired: 2 out]
        n223 = call "Variables.vi"("value"=w456, "Tag in"="laser.power.set", "Command"=T4."ChangeValue") -> ()  [unwired: 3 out]
      }
      event "Shutter": Value Change {
        n224 = event-data() -> ()  [unwired: 7 out]
        n225 = Select(t="1", s="Shutter", f="0") -> (s? t:f=w460:string)
        n226 = call "Variables.vi"("value"=w460, "Tag in"="laser.shutter.set" ("Name"), "Command"=T4."ChangeValue") -> ()  [unwired: 1 in, 2 out]
      }
      event Menu Selection (User) {
        # "run menu"
        n227 = event-data() -> ("ItemTag"=w470:string)  [unwired: 7 out]
        n228 = Search 1D Array(1D array=w469, element=w470) -> (index of element=w471:i32)  [unwired: 1 out]
        n229 = Index Array(array=w468, index=w471) -> (element=w472:refnum<vi>)
        n230 = case shown="\"Exit\"" w470 {
          tunnel: [FALSE TRUE FALSE] -> w467
          frame "True", Default {
            # "no special command"
          }
          frame "Exit" {
          }
          frame "Cancel" {
            n231 = call "Cancel.vi"() -> ()  [unwired: 1 out]
          }
        }
        n232 = Not A Number/Path/Refnum?(number/path/refnum=w472) -> (NaN/Path/Refnum?=w473:bool)
        n233 = case shown="False" w473 {
          tunnel: w472 -> [w478 _]
          tunnel: w470 -> [w477 _]
          frame False {
            n234 = call "OpenRunGUI.vi"("VI Refnum"=w478, "Menu"=w477) -> ()  [unwired: 1 out]
          }
          frame True {
            # "no vi defined\ne.g top level menu"
          }
        }
      }
      event Panel Close? {
        w480 = TRUE ("Discard?")
        n235 = event-data() -> ()  [unwired: 5 out]
        n236 = event-data("Discard?"=w480) -> ()  [unwired: 1 in, 1 out]
      }
    }
    "endGUI" <- w186
  }
  n237 = Release Notifier(notifier=w24) -> ()  [unwired: 1 in, 4 out]
  n238 = call "ImaqStorage.vi"("Number"=w21, "Command"=T5."DecreaseAccess") -> ()  [unwired: 1 in, 2 out]
  n239 = flat-sequence {
    tunnel: w2 -> [w482]
    tunnel: w1 -> [w481]
    frame #0 {
      n240 = call-poly <vilib>:"Close Input Device.vi"("device ID"=w482) -> ("error out"=w483:errorcluster)  [unwired: 1 in, 8 out]
      n241 = stacked-sequence {
        frame #0 {
          n242 = call "Variables.vi"("value"="show", "Tag in"="colibri.message", "Command"=T4."ChangeValue") -> ()  [unwired: 3 out]
        }
        frame #1 {
          n243 = Wait (ms)(milliseconds to wait=u32 500) -> ()  [unwired: 1 out]
        }
        frame #2 {
          n244 = call "Variables.vi"("value"="shutdown", "Tag in"="colibri.message", "Command"=T4."ChangeValue") -> ()  [unwired: 3 out]
        }
      }
      n245 = for {
        tunnel: w481 -> [w491] mode=indexing
        n246 = Not A Number/Path/Refnum?(number/path/refnum=w491) -> (NaN/Path/Refnum?=w492:bool)
        n247 = case shown="False" w492 {
          tunnel: w491 -> [w493 _]
          frame False {
            n248 = Close Reference(reference=w493) -> ()  [unwired: 1 in, 1 out]
          }
          frame True {
          }
        }
      }
      n249 = call <vilib>:"General Error Handler.vi"("error in (no error)"=w483) -> ()  [unwired: 1 in, 14 out]
      n250 = invoke class="VI" method="FP.Close"() -> ()  [unwired: 3 in, 3 out]
    }
  }
